vi "Write D.vi"(8 "error in (no error)":errorcluster, 10 "D":dbl, 11 "Change PID Controls MSG in":refnum<class "Change PID Controls MSG.lvclass">) -> (0 "error out":errorcluster, 3 "Change PID Controls MSG out":refnum<class "Change PID Controls MSG.lvclass">)   [LabVIEW 2014, in "Change PID Controls MSG.lvclass"]
uses:
  Change PID Controls MSG.lvclass
  Change PID Controls MSG.lvclass/Change PID Controls MSG.ctl
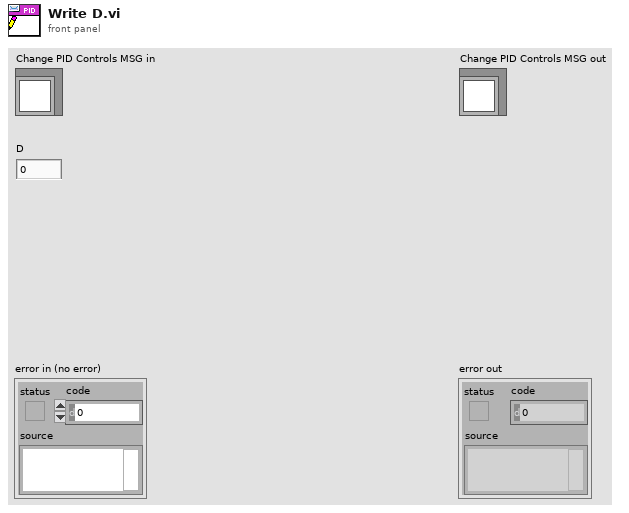
[diagram p1: front panel]
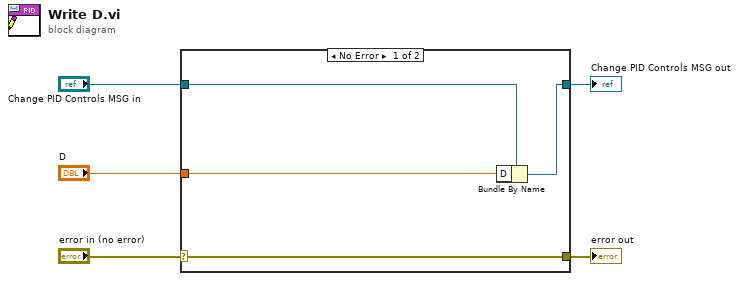
[diagram p0: block diagram]
diagram:
  n1 = case shown="No Error" "error in (no error)" {
    selector: "error in (no error)" -> [w9 w10]
    tunnel: [w9 w10] -> w4
    tunnel: [w7 w11] -> w2
    tunnel: "Change PID Controls MSG in" -> [w8 w11]
    tunnel: "D" -> [w6 _]
    frame No Error {
      n2 = Bundle By Name(cluster=w8, "D"=w6) -> (w7:refnum<class "Change PID Controls MSG.lvclass">)
    }
    frame Error {
    }
  }
  "error out" <- w4
  "Change PID Controls MSG out" <- w2
